vi "UpdatePasswordOfUserInDatabase.vi"(8 "error in (no error)":errorcluster, 9 "User ID":string, 10 "DatabaseConnectionInfo":T1, 11 "New password":string) -> (0 "error out":errorcluster)   [LabVIEW 2017]
uses:
  <vilib>/addons/database/Connection.llb/DB Tools Open Connec (Path).vi
  <vilib>/addons/database/NI_Database_API.lvlib
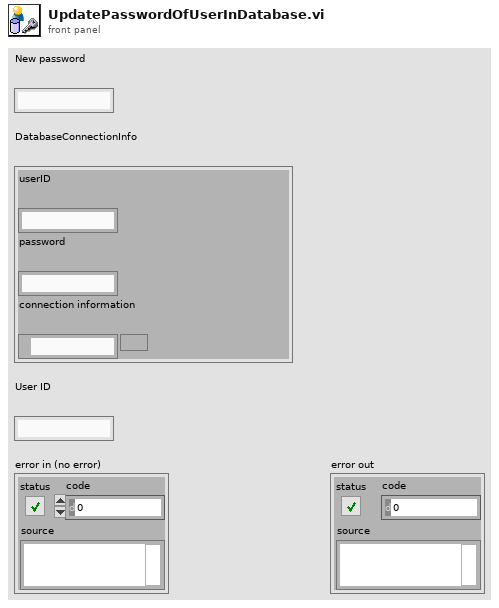
[diagram p1: front panel]
types:
  T1 = cluster{"userID":string, "password":string, "connection information":path}
  T2 = typedef "NI_Database_API.lvlib/Conn ObjectReference.ctl" = refnum<k1>
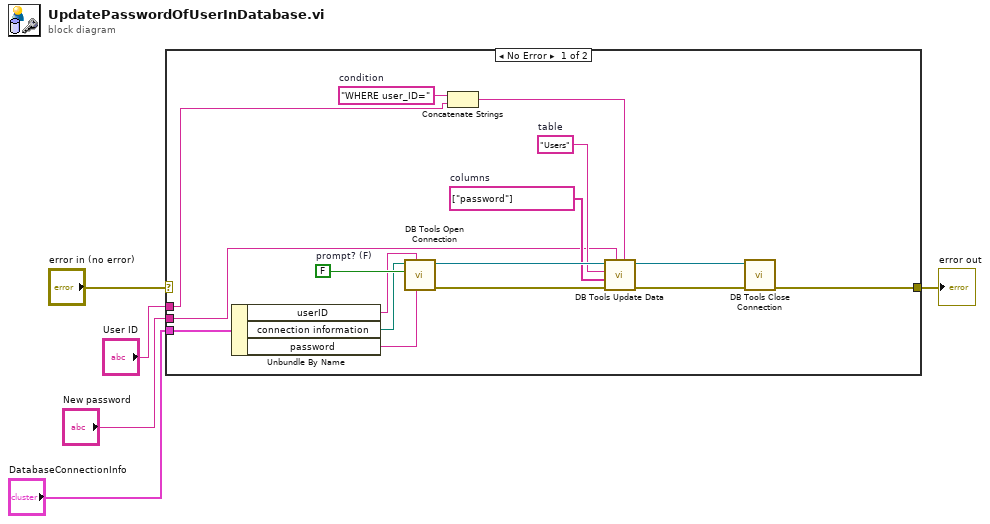
[diagram p0: block diagram]
diagram:
  n1 = case shown="No Error" "error in (no error)" {
    selector: "error in (no error)" -> [_ w22]
    tunnel: [w21 w22] -> w3
    tunnel: "User ID" -> [w12 _]
    tunnel: "New password" -> [w10 _]
    tunnel: "DatabaseConnectionInfo" -> [w9 _]
    frame No Error {
      w13 = "WHERE user_ID="  # condition
      w14 = string[] ["password"]  # columns
      w15 = "Users"  # table
      w20 = FALSE  # prompt? (F)
      n2 = Unbundle By Name(w9) -> ("userID"=w8:string, "connection information"=w6:path, "password"=w7:string)
      n3 = call-poly <vilib>:"DB Tools Open Connection.vi"("password"=w7, "userID"=w8, "prompt? (F)"=w20, "connection information"=w6) -> ("error out"=w18:errorcluster, "connection reference"=w19:T2)  [unwired: 4 in]
      n4 = Concatenate Strings(w13, w12) -> (w11:string)
      n5 = call <vilib>:"DB Tools Update Data.vi"("condition"=w11, "data"=w10, "error in (no error)"=w18, "columns"=w14, "table"=w15, "connection reference"=w19) -> ("error out"=w17:errorcluster, "connection reference out"=w16:T2)  [unwired: 4 in]
      n6 = call <vilib>:"DB Tools Close Connection.vi"("error in (no error)"=w17, "connection reference"=w16) -> ("error out"=w21:errorcluster)  [unwired: 5 in]
    }
    frame Error {
    }
  }
  "error out" <- w3
